vi "Controllo coppia.vi"(0 "C attuale":dbl, 1 "fine rampa C in":bool, 2 "Tutti i dati":T2, 3 "Coppia":T8, 4 "Cmax RPMmax\n inverter":cluster{"Vel max(RPM)":dbl, "Cmax (nm)":dbl}, 5 "RPM PROVA":refnum<vi>, 6 "Coppia letta tors":dbl, 7 "Reset comp":bool, 8 "COPPIA DI FRENATURA [Nm]":refnum<vi>, 9 "Forza controllo vel":bool, 10 "Set C":dbl, 11 "Fine rampa F":bool, 12 "Cmax":dbl, 13 "LOOP TIME (ms)":u32) -> (14 "fine rampa C out":bool, 15 "C stabile":bool, 16 "Set C out":dbl, 17 "Out C":dbl, 18 "Tempo rampa (s)":dbl)   [LabVIEW 2019]
uses:
  cDAQ_PLC Folder/cDAQ/AO List.ctl
  cDAQ_PLC Folder/cDAQ/SET SINGLE AO.ctl
  cDAQ_PLC Folder/cDAQ/DO List.ctl
  cDAQ_PLC Folder/cDAQ/SET SINGLE DO.ctl
  Global FINE AVVIO.vi
  Global_Cmecc_RotBlocc.vi
  <vilib>/addons/control/pid/NI_PID_pid.lvlib
  Global set coppia.vi
  Global stato ctrl coppia.vi
  Global prova in corso.vi
  Global_scelta_banco.vi
  Global Stop command.vi
  Global ctrl potenza.vi
  Servo avviamento.vi
  <vilib>/Analysis/NI_AALBase.lvlib
  <vilib>/addons/control/pid/pid.llb/PID (DBL).vi
  <vilib>/Analysis/1siggen.llb/Ramp Pattern by Samples.vi
  cDAQ/LettureCDAQ_PLC.ctl
  controls/statoAO_plc.ctl
  controls/statoDO.ctl
  ST1200_LIST_IO/StatoDO_PLC.ctl
  cDAQ_PLC Folder/controls/StatoAO_cdaq.ctl
  controls/Tutti_i_dati.ctl
panel:
  out "Boolean":bool=TRUE
  out "Ramp":dbl[](array[numeric])
  in  "Periodo set rpm[s] b2":dbl=2.0 format="%#_13g"
  in  "step rpm B2":dbl=0.5 format="%#_13g"
  in  "Nm b2":dbl=2.0 format="%#_13g"
  in  "Precisione b2":dbl=0.2
  in  "Nm b1":dbl=0.015 format="%#_13g"
  in  "Precisione b1":dbl=0.01
  out "s? t:f":string
  in  "PID b2 gains ctrl velocità":T1={"proportional gain (Kc)"=5.0, "integral time (Ti, min)"=0.01, "derivative time (Td, min)"=0.0}
  out "fine rampa":bool
  in  "reinitialize? (F)":bool
  in  "PID b1 gains ctrl velocità":T1={"proportional gain (Kc)"=250.0, "integral time (Ti, min)"=0.003, "derivative time (Td, min)"=0.0} {"derivative time (Td, min)" format="%.3f"; "integral time (Ti, min)" format="%.3f"; "proportional gain (Kc)" format="%.3f"}
  out "x < y?":bool
  out "x > y?":bool
  in  "step rpm B1":dbl=2.0 format="%#_13g"
  in  "max variazione rpm":dbl=2300.0 format="%#_13g"
  in  "Periodo set rpm[s] b1":dbl=0.5 format="%#_13g"
  out "RPM iniziali":dbl
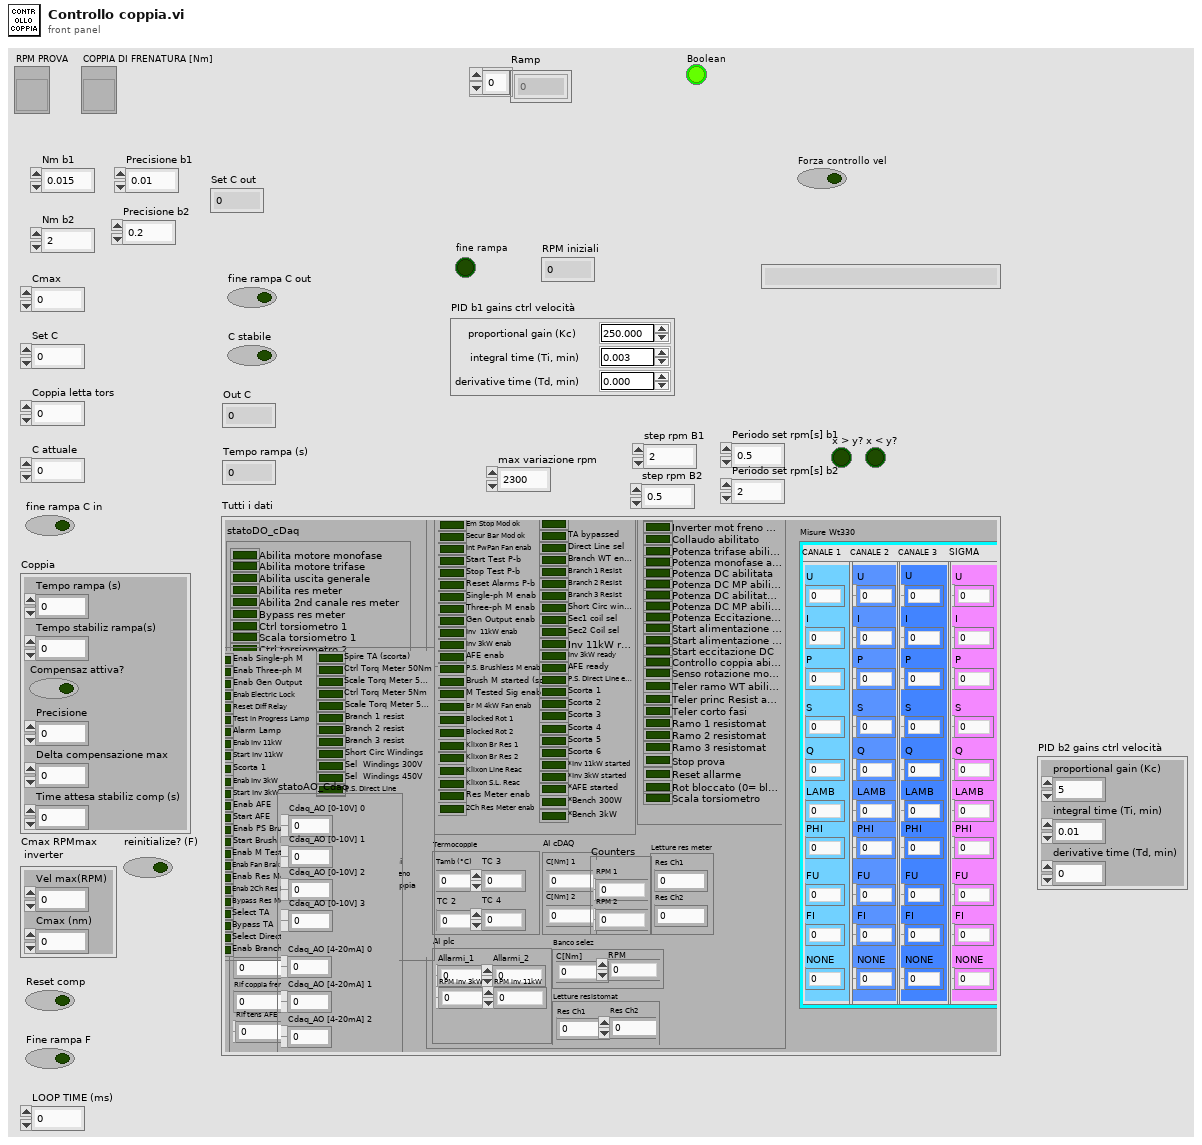
[diagram p1: front panel]
types:
  T1 = cluster{"proportional gain (Kc)":dbl, "integral time (Ti, min)":dbl, "derivative time (Td, min)":dbl}
  T2 = typedef "Tutti_i_dati.ctl" = cluster{"Letture":T3, "Misure Wt330":cluster{"CANALE 1":cluster{"U":dbl, "I":dbl, "P":dbl, "S":dbl, "Q":dbl, "LAMB":dbl, "PHI":dbl, "FU":dbl, "FI":dbl, "NONE":dbl}, "CANALE 2":cluster{"U":dbl, "I":dbl, "P":dbl, "S":dbl, "Q":dbl, "LAMB":dbl, "PHI":dbl, "FU":dbl, "FI":dbl, "NONE":dbl}, "CANALE 3":cluster{"U":dbl, "I":dbl, "P":dbl, "S":dbl, "Q":dbl, "LAMB":dbl, "PHI":dbl, "FU":dbl, "FI":dbl, "NONE":dbl}, "SIGMA":cluster{"U":dbl, "I":dbl, "P":dbl, "S":dbl, "Q":dbl, "LAMB":dbl, "PHI":dbl, "FU":dbl, "FI":dbl, "NONE":dbl}}, "statoAO_PLC":T4, "statoDO_cDaq":T5, "StatoDO_PLC":T6, "statoAO_Cdaq":T7}
  T3 = typedef "LettureCDAQ_PLC.ctl" = cluster{"DI-logici":cluster{"Sistema OK":bool, "Inverter mot freno Run":bool, "Collaudo abilitato":bool, "Potenza trifase abilitata":bool, "Potenza monofase abilitata":bool, "Potenza DC abilitata":bool, "Potenza DC MP abilitata":bool, "Potenza DC abilitata no WT":bool, "Potenza DC MP abilitata no WT":bool, "Potenza Eccitazione abilitata":bool, "Start alimentazione AC":bool, "Start alimentazione DC":bool, "Start eccitazione DC":bool, "Controllo coppia abilitato":bool, "Senso rotazione motore freno":bool, "Teler ramo WT abilitato":bool, "Teler princ Resist abilitato":bool, "Teler corto fasi":bool, "Ramo 1 resistomat":bool, "Ramo 2 resistomat":bool, "Ramo 3 resistomat":bool, "Stop prova":bool, "Reset allarme":bool, "Rot bloccato (0= bloccato)":bool, "Scala torsiometro":bool}, "Termocoppie":cluster{"Tamb (°C)":dbl, "TC 2":dbl, "TC 3":dbl, "TC 4":dbl}, "AI cDAQ":cluster{"C[Nm] 1":dbl, "C[Nm] 2":dbl}, "Counters":cluster{"RPM 1":dbl, "RPM 2":dbl}, "Stato DI_Cdaq":cluster{"Motore monofase abil":bool, "Motore trifase abil":bool, "Uscita generale abil":bool, "2nd ch res meter abil":bool, "TA selezionati":bool, "Pulsante Start prova":bool, "Pulsante Stop prova":bool, "Pulsante Reset allarmi":bool, "Secondari TA aperti":bool, "Res meter abil":bool, "Scorta 1":bool, "Scorta 2":bool, "Scorta 3":bool, "Scorta 4":bool, "Scorta 5":bool, "Scorta 6":bool, "Scorta 7":bool, "Scorta 8":bool, "Scorta 9":bool, "Scorta 10":bool, "Scorta 11":bool, "Scorta 12":bool, "Scorta 13":bool, "Scorta 14":bool, "Scorta 15":bool, "Scorta 16":bool, "Scorta 17":bool, "Scorta 18":bool, "Scorta 19":bool, "Scorta 20":bool, "Scorta 21":bool, "Scorta 22":bool}, "Stato DI_PLC":cluster{"Diff Relay On":bool, "Em Stop Mod ok":bool, "Secur Bar Mod ok":bool, "Int PwPan Fan enab":bool, "Start Test P-b":bool, "Stop Test P-b":bool, "Reset Alarms P-b":bool, "Single-ph M enab":bool, "Three-ph M enab":bool, "Gen Output enab":bool, "Inv  11kW enab":bool, "Inv 3kW enab":bool, "AFE enab":bool, "P.S. Brushless M enab":bool, "Brush M started (scorta)":bool, "M Tested Sig enab":bool, "Br M 4kW Fan enab":bool, "Blocked Rot 1":bool, "Blocked Rot 2":bool, "Klixon Br Res 1":bool, "Klixon Br Res 2":bool, "Klixon Line Reac":bool, "Klixon S.L. Reac":bool, "Res Meter enab":bool, "2Ch Res Meter enab":bool, "Bypass Res Meter":bool, "TA selected":bool, "TA bypassed":bool, "Direct Line sel":bool, "Branch WT enab":bool, "Branch 1 Resist":bool, "Branch 2 Resist":bool, "Branch 3 Resist":bool, "Short Circ windings":bool, "Sec1 coil sel":bool, "Sec2 Coil sel":bool, "Inv 11kW ready":bool, "Inv 3kW ready":bool, "AFE ready":bool, "P.S. Direct Line enab":bool, "Scorta 1":bool, "Scorta 2":bool, "Scorta 3":bool, "Scorta 4":bool, "Scorta 5":bool, "Scorta 6":bool, "*Inv 11kW started":bool, "*Inv 3kW started":bool, "*AFE started":bool, "*Bench 300W":bool, "*Bench 3kW":bool}, "Letture res meter":cluster{"Res Ch1":dbl, "Res Ch2":dbl}, "Banco selez":cluster{"C[Nm]":dbl, "RPM":dbl}, "AI plc":cluster{"Allarmi_1":dbl, "Allarmi_2":dbl, "RPM inv 3kW":dbl, "RPM inv 11kW":dbl}, "Letture resistomat":cluster{"Res Ch1":dbl, "Res Ch2":dbl}}
  T4 = typedef "statoAO_plc.ctl" = cluster{"Rif vel freno":dbl, "Rif coppia freno":dbl, "Rif tens AFE":dbl, "Rif freq AFE":dbl}
  T5 = typedef "statoDO.ctl" = cluster{"Abilita motore monofase":bool, "Abilita motore trifase":bool, "Abilita uscita generale":bool, "Abilita res meter":bool, "Abilita 2nd canale res meter":bool, "Bypass res meter":bool, "Ctrl torsiometro 1":bool, "Scala torsiometro 1":bool, "Ctrl torsiometro 2":bool, "Scala torsiometro 2":bool, "Seleziona TA":bool, "Seleziona linea diretta":bool, "Seleziona spire TA":bool, "Bypass TA":bool, "Lampada Test in progress":bool, "Lampada allarme":bool, "Apri TA secondari":bool, "Scorta 1":bool, "Scorta 2":bool, "Scorta 3":bool, "Scorta 4":bool, "Scorta 5":bool, "Scorta 6":bool, "Scorta 7":bool, "Scorta 8":bool, "Scorta 9":bool, "Scorta 10":bool, "Scorta 11":bool, "Scorta 12":bool, "Scorta 13":bool, "Scorta 14":bool, "Scorta 15":bool}
  T6 = typedef "StatoDO_PLC.ctl" = cluster{"Enab Single-ph M":bool, "Enab Three-ph M":bool, "Enab Gen Output":bool, "Enab Electric Lock":bool, "Reset Diff Relay":bool, "Test in Progress Lamp":bool, "Alarm Lamp":bool, "Enab Inv 11kW":bool, "Start Inv 11kW":bool, "Scorta 1":bool, "Enab Inv 3kW":bool, "Start Inv 3kW":bool, "Enab AFE":bool, "Start AFE":bool, "Enab PS Brush M":bool, "Start Brush M (scorta)":bool, "Enab M Tested Sig":bool, "Enab Fan Brak M 4kW":bool, "Enab Res Meter":bool, "Enab 2Ch Res Meter":bool, "Bypass Res Meter":bool, "Select TA":bool, "Bypass TA":bool, "Select Direct Line":bool, "Enab Branch WT":bool, "Spire TA (scorta)":bool, "Ctrl Torq Meter 50Nm":bool, "Scale Torq Meter 50Nm ":bool, "Ctrl Torq Meter 5Nm":bool, "Scale Torq Meter 5Nm":bool, "Branch 1 resist":bool, "Branch 2 resist":bool, "Branch 3 resist":bool, "Short Circ Windings":bool, "Sel  Windings 300V":bool, "Sel  Windings 450V":bool, "P.S. Direct Line":bool, "Scorta 2":bool, "Scorta 3":bool, "Scorta 4":bool, "Scorta 5":bool, "Scorta 6":bool, "*Reset Allarmi":bool, "*Senso Rotaz freno":bool, "*Controllo Coppia":bool, "*Abilita freno":bool, "*Marcia freno":bool, "*Watch dog":bool, "*Bench 300W":bool, "*Bench 3kW":bool}
  T7 = typedef "StatoAO_cdaq.ctl" = cluster{"Cdaq_AO [0-10V] 0":dbl, "Cdaq_AO [0-10V] 1":dbl, "Cdaq_AO [0-10V] 2":dbl, "Cdaq_AO [0-10V] 3":dbl, "Cdaq_AO [4-20mA] 0":dbl, "Cdaq_AO [4-20mA] 1":dbl, "Cdaq_AO [4-20mA] 2":dbl, "Cdaq_AO [4-20mA] 3":dbl, "Cdaq_AO [4-20mA] 4":dbl, "Cdaq_AO [4-20mA] 5":dbl, "Cdaq_AO [4-20mA] 6":dbl, "Cdaq_AO [4-20mA] 7":dbl}
  T8 = cluster{"Tempo rampa (s)":dbl, "Tempo stabiliz rampa(s)":dbl, "Compensaz attiva?":bool, "Precisione":dbl, "Delta compensazione max":dbl, "Time attesa stabiliz comp (s)":dbl}
  T9 = typedef "SET SINGLE AO.ctl" = cluster{"AO":T10, "Value":dbl}
  T10 = typedef "AO List.ctl" = enum16{"OFF: ALL AO", "Vout Variac", "Vout Freq", "Vout 3", "Vout 4", "Forza AO", "*V eccitazion", "*I eccitazione", "*Rif vel inv freno", "*Rif coppia inv freno", "Exit"}
  T11 = enum8{"Enabled", "Disabled", "Disabled and Grayed Out"}
  T12 = typedef "SET SINGLE DO.ctl" = cluster{"DO":T13, "Value":bool}
  T13 = typedef "DO List.ctl" = enum16{"OFF: ALL DO", "Seleziona banco 1", "Seleziona banco 2", "Reset allarmi", "*Start inverter motore freno", "*Senso rotaz motore freno", "*Abilitazione controllo coppia", "Bypass res meter", "Telerutt scelta linea 60A", "Telerutt scelta spire 50A", "Scelta TA", "Bypass TA", "*Abilit teler ramo WT", "*Abil teler ramo princ Resist", "*Abil teler ramo 1 Resist", "*Abil teler ramo 2 Resist", "*Abil teler ramo 3 Resist", "*Abil cortocirc avvolgim", "*Controllo torsiometro", "*Scala torsiometro", "Collaudo in corso", "*Allarme presente", "Abilita piattaf (0=abil)", "Abilitazione elettroserratura", "Exit", "*Abilita collaudo", "*Abilita potenza trifase", "*Abilita potenza monofase", "*Abilita potenza DC", "*Abilita potenza DC no WT", "*Abilita potenza DC MP", "*Abilita potenza DC MP no WT", "*Start Alimentazione AC", "*Start Alimentazione DC", "*Start eccitazione DC", "*Disabilita teleruttori potenza", "Set teleruttori prova a freddo", "Watchdog", "Forza DO", "*Abil teler ramo princ ResistMeter", "Abil AFE rigenerativo"}
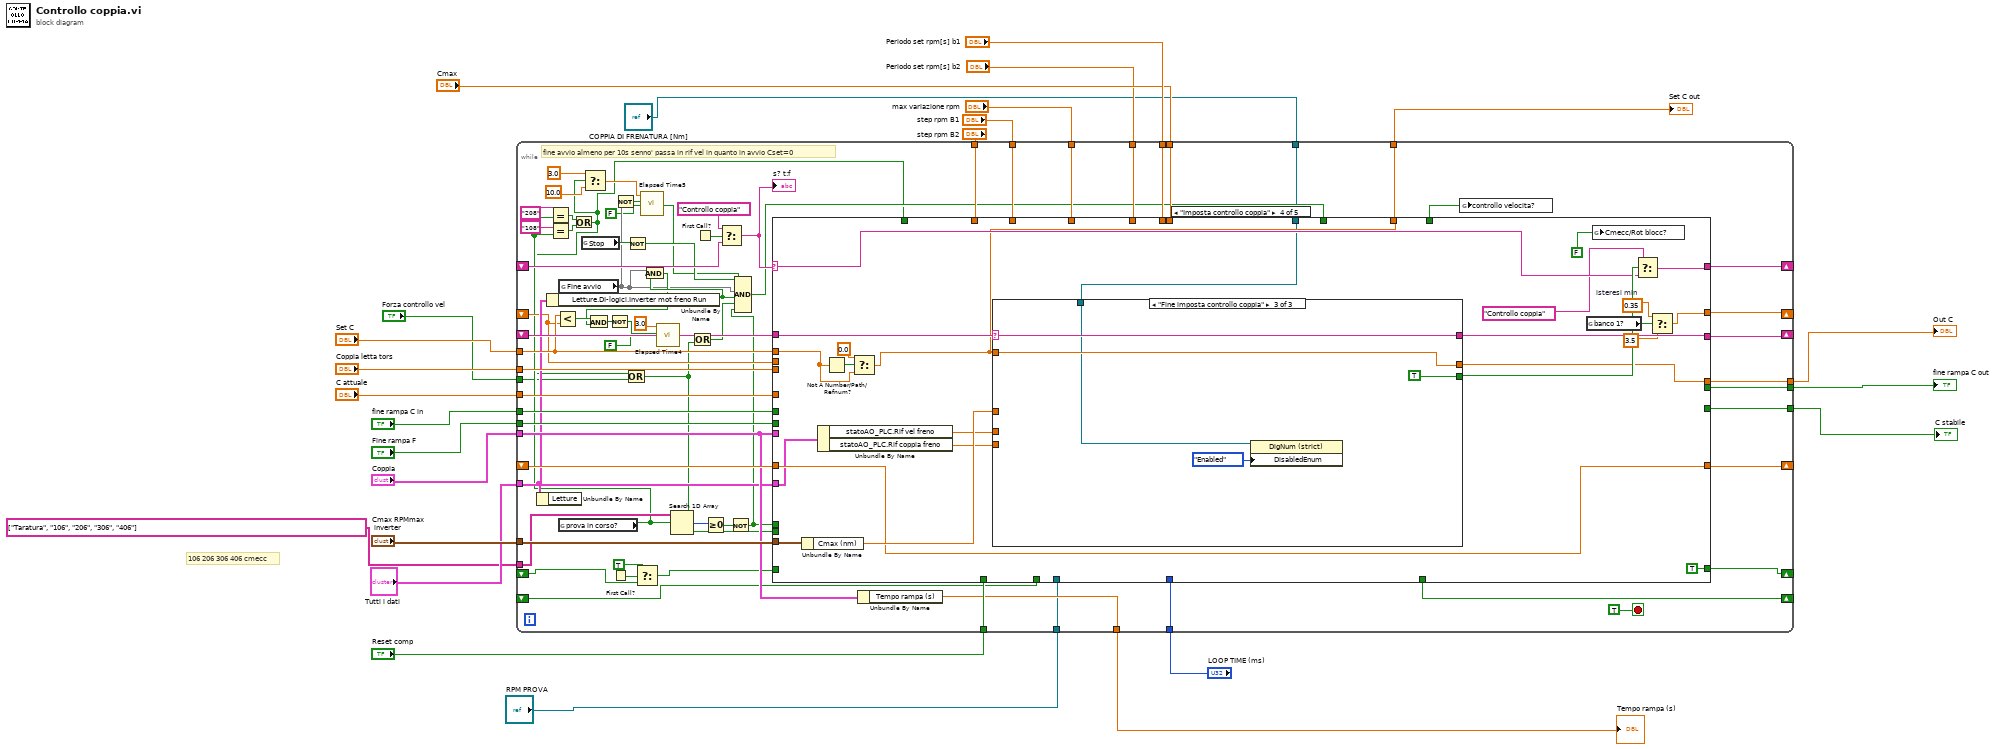
[diagram p0: block diagram]
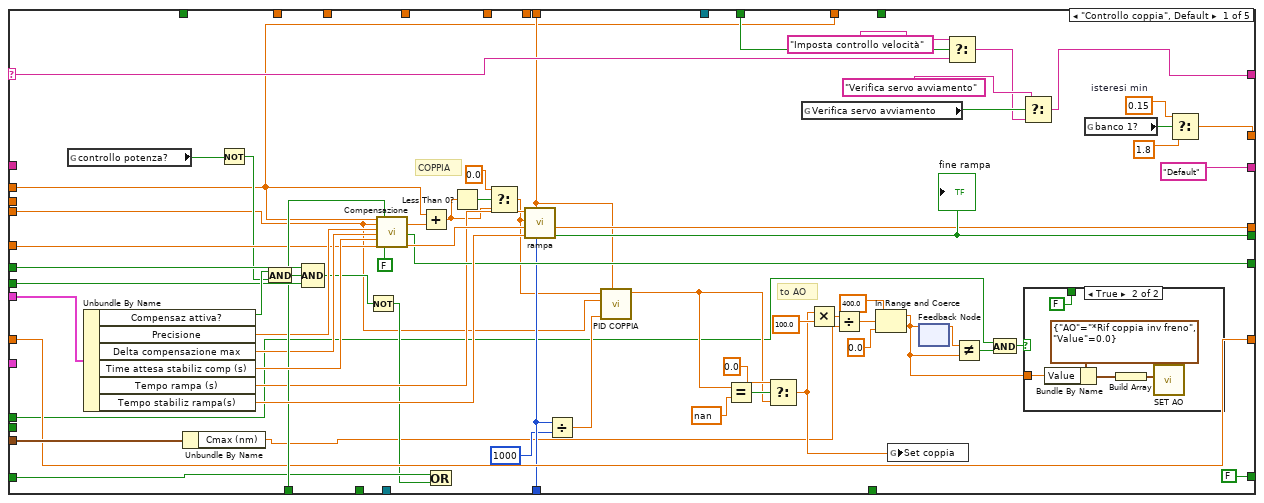
[diagram p2: hidden frame]
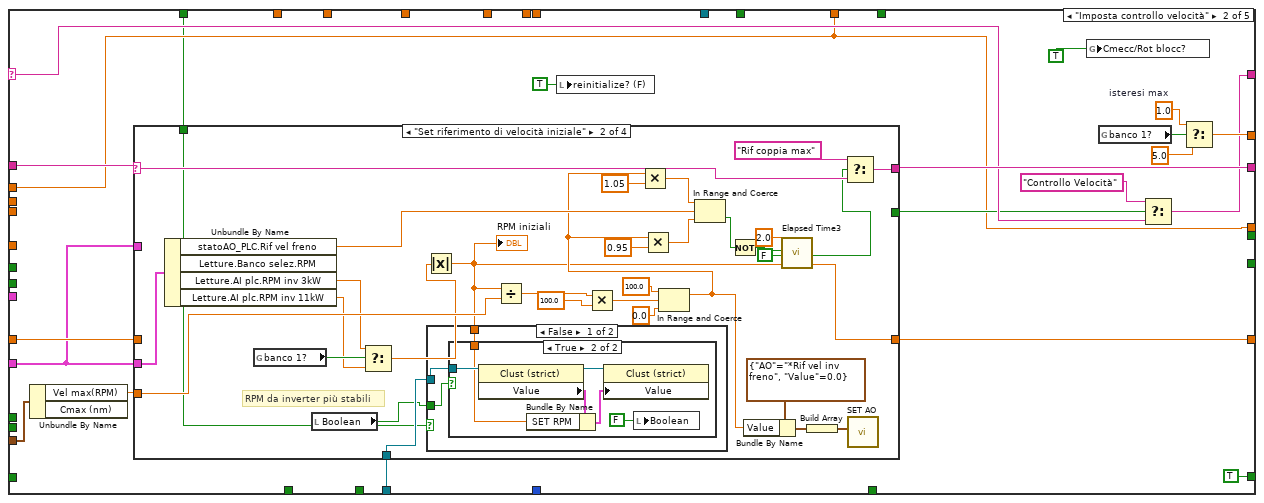
[diagram p4: hidden frame]
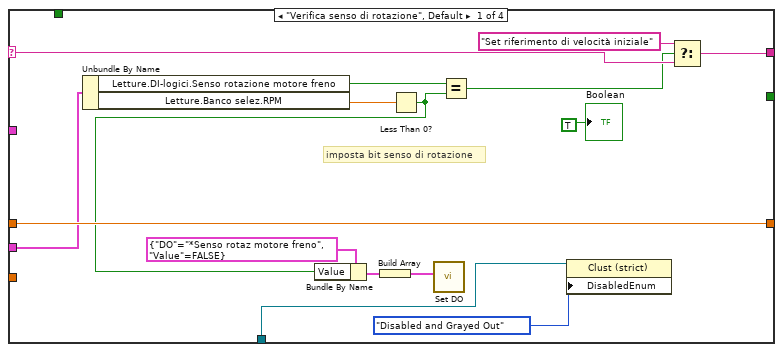
[diagram p5: hidden frame]
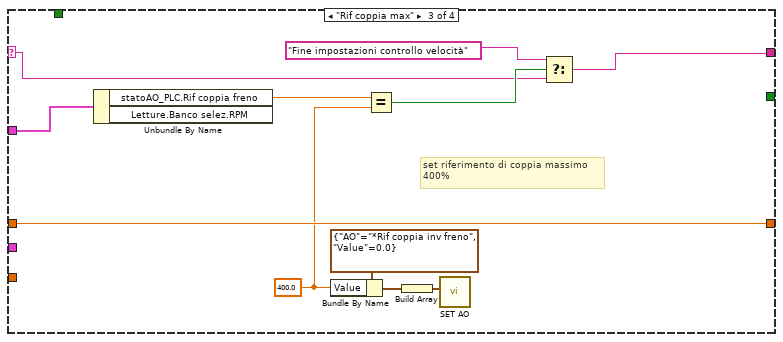
[diagram p8: hidden frame]
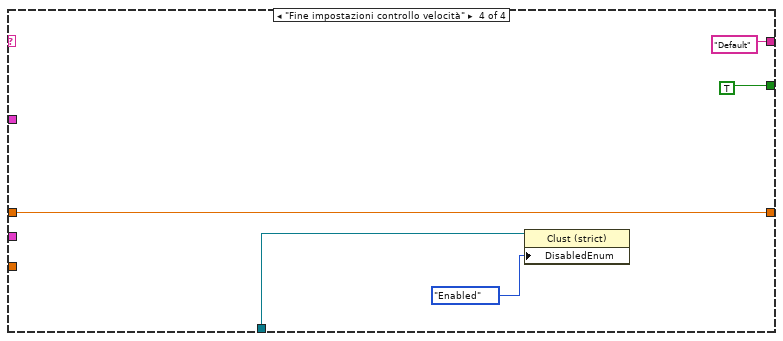
[diagram p9: hidden frame]
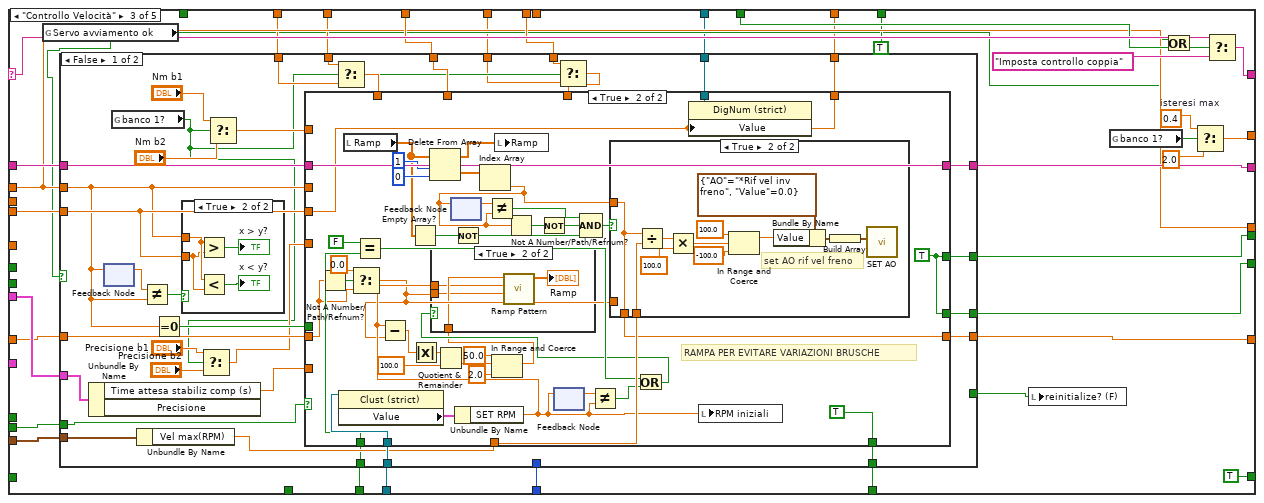
[diagram p10: hidden frame]
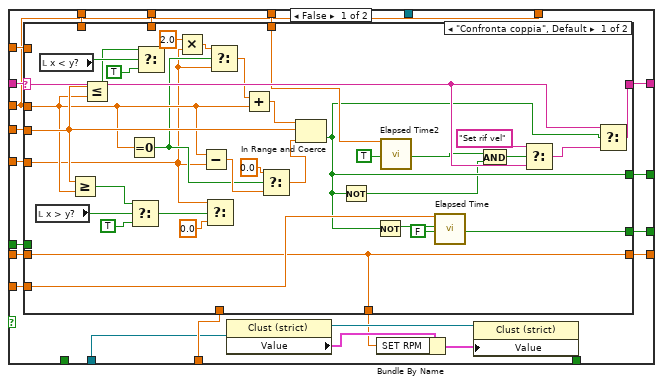
[diagram p11: hidden frame]
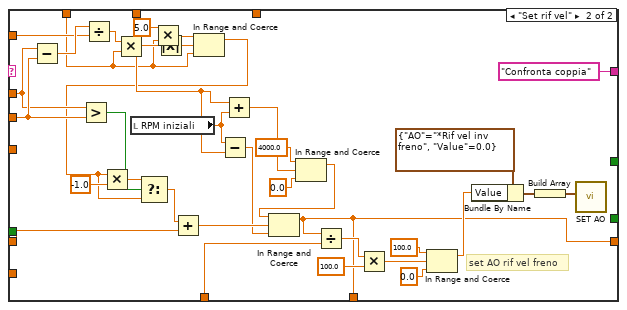
[diagram p12: hidden frame]
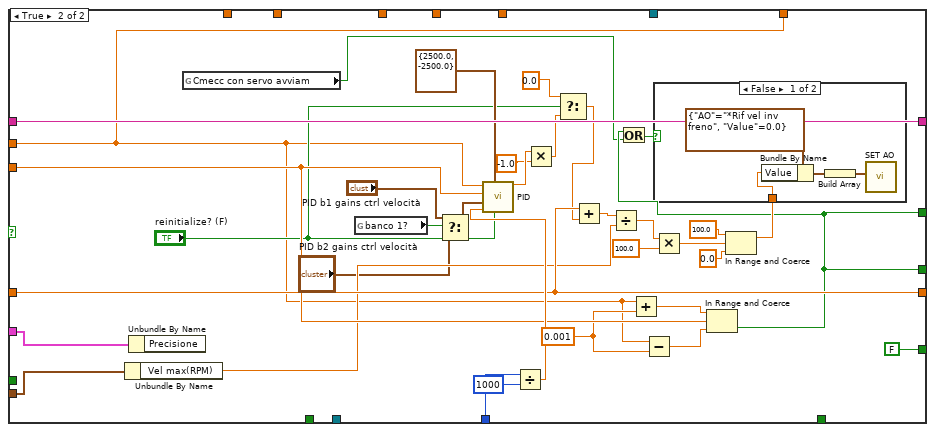
[diagram p16: hidden frame]
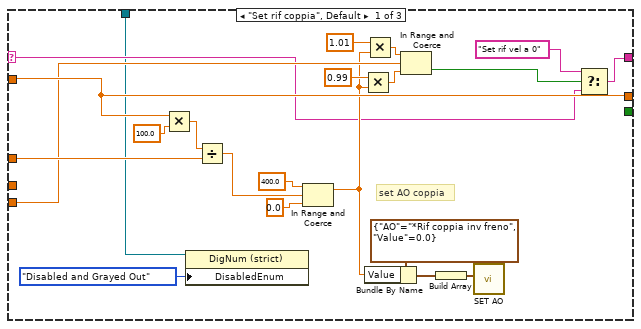
[diagram p18: hidden frame]
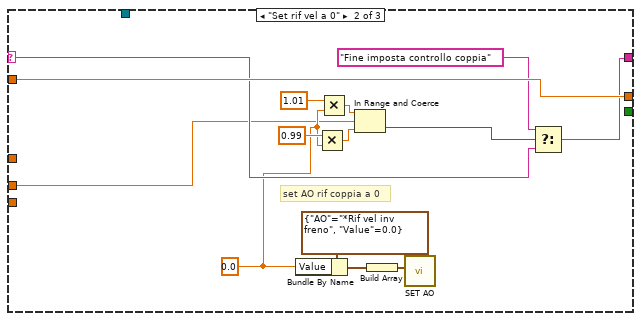
[diagram p19: hidden frame]
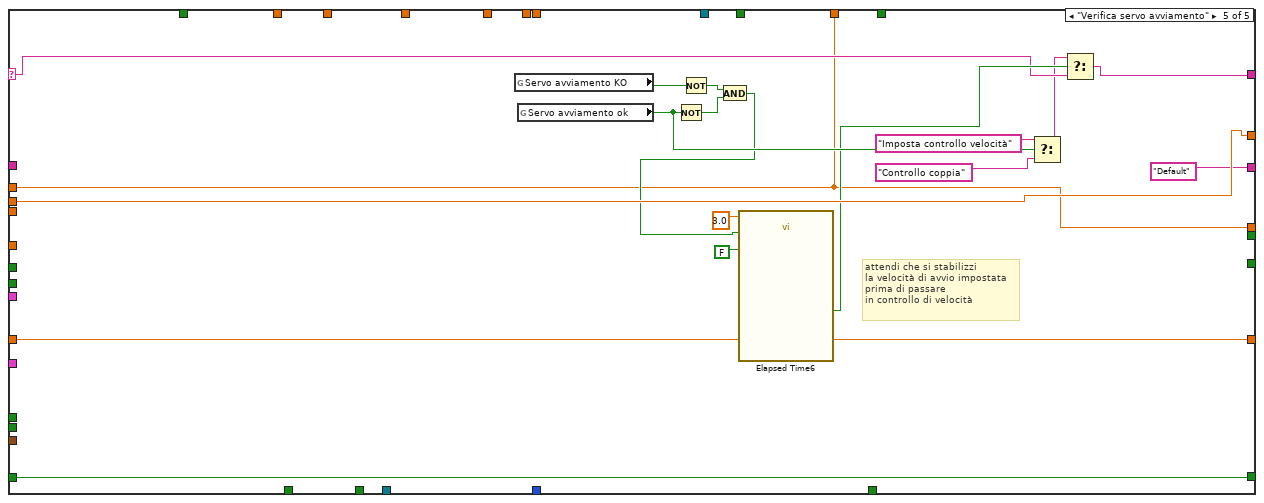
[diagram p20: hidden frame]
diagram:
  # "106 206 306 406 cmecc"
  n1 = while {
    tunnel: "LOOP TIME (ms)" -> [w99]
    tunnel: "C attuale" -> [w98]
    tunnel: "Coppia" -> [w79]
    tunnel: "fine rampa C in" -> [w97]
    tunnel: "Fine rampa F" -> [w96]
    tunnel: "Reset comp" -> [w95]
    tunnel: "Coppia letta tors" -> [w94]
    tunnel: "Set C" -> [w75]
    tunnel: [w93] -> w22
    tunnel: [w92] -> w23
    tunnel: [w78] -> w24
    tunnel: "Cmax RPMmax\n inverter" -> [w91]
    tunnel: [w90] -> w14
    tunnel: "Cmax" -> [w89]
    shift-right: [w87] -> _
    shift-left: _ -> [w77]
    shift-right: [w85] -> _
    shift-left: _ -> [w86]
    tunnel: "Tutti i dati" -> [w70]
    shift-right: [w84] -> _
    shift-left: _ -> [w83]
    tunnel: "max variazione rpm" -> [w82]
    tunnel: "step rpm B1" -> [w81]
    tunnel: "Periodo set rpm[s] b1" -> [w80]
    tunnel: string[] ["Taratura", "106", "206", "306", "406"] -> [w69]
    shift-right: [w61] -> _
    shift-left: _ -> [w47]
    shift-right: [w55] -> _
    shift-left: _ -> [w53]
    tunnel: "step rpm B2" -> [w50]
    tunnel: "Periodo set rpm[s] b2" -> [w45]
    tunnel: "Forza controllo vel" -> [w29]
    tunnel: "RPM PROVA" -> [w41]
    tunnel: [w40] -> w3
    shift-right: [w39] -> _
    shift-left: _ -> [w38]
    tunnel: "COPPIA DI FRENATURA [Nm]" -> [w26]
    stop <- TRUE stop-if-true
    # "fine avvio almeno per 10s senno' passa in rif vel in quanto in avvio Cset=0"
    n2 = Unbundle By Name(w70) -> ()  [unwired: 1 out]
    n3 = Unbundle By Name(w70) -> ("Letture.DI-logici.Inverter mot freno Run"=w64:bool)
    n4 = Less?(x=w75, y=w47) -> (x < y?=w73:bool)
    n5 = global read "Global prova in corso.vi" "prova in corso?"() -> (w34:bool)
    n6 = Equal?(x=w34, y="208") -> (x = y?=w30:bool)
    n7 = Equal?(x="108", y=w34) -> (x = y?=w31:bool)
    n8 = global read "Global fine avvio.vi" "Fine avvio"() -> (w60)
    n9 = Or(x=w30, y=w31) -> (x .or. y?=w27:bool)
    n10 = global read "Global Stop command.vi" "Stop"() -> (w66:bool)
    n11 = Select(t=3.0, s=w27, f=10.0 ("Time Target (s)")) -> (s? t:f=w36:dbl)
    n12 = First Call?() -> (First Call?: T/F=w54:bool)
    n13 = Not(x=w60) -> (.not. x?=w59:bool)
    n14 = Or(x=w27, y=w29) -> (x .or. y?=w28:bool)
    n15 = Not(x=w66) -> (.not. x?=w65:bool)
    n16 = Select(t=TRUE, s=w54, f=w53) -> (s? t:f=w52:bool)
    n17 = call "Elapsed Time5"("Time Target (s)"=w36, "Reset"=w59, "Auto Reset"=FALSE) -> ("Time has Elapsed"=w57:bool)  [unwired: 9 in, 7 out]
    n18 = And(x=w60, y=w64) -> (x .and. y?=w62:bool)
    n19 = And(x=w73, y=w62) -> (x .and. y?=w63:bool)
    n20 = Not(x=w63) -> (.not. x?=w72:bool)
    n21 = call "Elapsed Time4"("Time Target (s)"=3.0, "Reset"=w72, "Auto Reset"=FALSE) -> ("Time has Elapsed"=w43:bool)  [unwired: 9 in, 7 out]
    n22 = Search 1D Array(1D array=w69, element=w34) -> (index of element=w68:i32)  [unwired: 1 in]
    n23 = Or(x=w43, y=w28) -> (x .or. y?=w42:bool)
    n24 = First Call?() -> (First Call?: T/F=w56:bool)
    n25 = Greater Or Equal To 0?(x=w68) -> (x >= 0?=w67:bool)
    n26 = Select(t="Controllo coppia", s=w56, f=w77) -> (s? t:f=w48:string)
    "s? t:f" <- w48
    n27 = Not(x=w67) -> (.not. x?=w46:bool)
    n28 = Compound Arithmetic op=AND(w57, w65, w60, w64, w42, w46) -> (w44:bool)
    n29 = case shown="\"Imposta controllo coppia\"" w48 {
      selector: w48 -> [w139 w187 w292 w540 w589]
      tunnel: w99 -> [w134 _ w280 _ _]
      tunnel: w98 -> [w129 _ _ _ _]
      tunnel: w79 -> [w159 _ w290 _ _]
      tunnel: w97 -> [w158 _ _ _ _]
      tunnel: w96 -> [w156 _ _ _ _]
      tunnel: w95 -> [w155 _ _ _ _]
      tunnel: w94 -> [w111 _ w281 _ _]
      tunnel: w75 -> [w100 w170 w282 w524 w587]
      tunnel: [w132 _ w284 _ _] -> w93
      tunnel: [w153 _ w285 _ _] -> w92
      tunnel: w91 -> [w148 w185 w287 w544 _]
      tunnel: [w112 w170 w282 w537 w587] -> w90
      tunnel: w89 -> [w101 _ _ _ _]
      tunnel: [w104 w172 w293 w539 w595] -> w87
      tunnel: w44 -> [w138 _ w291 _ _]
      tunnel: w86 -> [_ w189 w296 w545 _]
      tunnel: ["Default" w188 w295 w542 "Default"] -> w85
      tunnel: w70 -> [_ w180 _ w534 _]
      tunnel: [w135 w182 w288 w536 w604] -> w84
      tunnel: w83 -> [w135 w181 w289 w536 w604]
      tunnel: w82 -> [_ _ w286 _ _]
      tunnel: w81 -> [_ _ w272 _ _]
      tunnel: w80 -> [_ _ w283 _ _]
      tunnel: [_ _ TRUE _ _] -> w76
      tunnel: [w125 w174 w275 w529 w602] -> w61
      tunnel: [FALSE TRUE TRUE TRUE w603] -> w55
      tunnel: w52 -> [w117 _ _ _ w603]
      tunnel: w50 -> [_ _ w271 _ _]
      tunnel: w47 -> [_ _ _ _ w602]
      tunnel: w46 -> [w102 _ _ _ _]
      tunnel: w45 -> [_ _ w268 _ _]
      tunnel: w41 -> [_ w171 w266 _ _]
      tunnel: w28 -> [_ _ w267 _ _]
      tunnel: [w100 w170 w265 w523 w587] -> w40
      tunnel: [_ _ w264 _ _] -> w39
      tunnel: w38 -> [_ _ w263 _ _]
      tunnel: w27 -> [_ w169 _ _ _]
      tunnel: w26 -> [_ _ w262 w522 _]
      frame "Controllo coppia", Default {
        w128 = 0.15  # isteresi min
        # "to AO"
        # "COPPIA"
        n30 = global read "Global ctrl potenza.vi" "controllo potenza?"() -> (w116:bool)
        n31 = Unbundle By Name(w159) -> ("Compensaz attiva?"=w157:bool, "Precisione"=w154:dbl, "Delta compensazione max"=w131:dbl, "Time attesa stabiliz comp (s)"=w160:dbl, "Tempo rampa (s)"=w151:dbl, "Tempo stabiliz rampa(s)"=w161:dbl)
        n32 = Unbundle By Name(w148) -> ("Cmax (nm)"=w113:dbl)
        n33 = Not(x=w116) -> (.not. x?=w123:bool)
        n34 = And(x=w157, y=w123) -> (x .and. y?=w124:bool)
        n35 = Compound Arithmetic op=AND(w158, w124, w156) -> (w115:bool)
        n36 = Not(x=w115) -> (.not. x?=w114:bool)
        n37 = call "Compensazione.vi"("Grandezza target"=w100, "Grandezza reale letta"=w111, "Precisione"=w154, "Delta compensazione max"=w131, "Time attesa stabilizzazione (s)"=w160, "Grandezza attuale in"=w129, "Reset comp?"=w155, "Compensazione abilitata"=FALSE) -> ("compensazione"=w162:dbl, "Grandezza stabilizz?"=w153:bool, "Grandezza attuale out"=w163:dbl)  [unwired: 9 in]
        n38 = Add(x=w100, y=w162) -> (x+y=w142:dbl)
        n39 = Or(x=w117, y=w114) -> ()  [unwired: 1 out]
        n40 = Less Than 0?(x=w142) -> (x < 0?=w143:bool)
        n41 = Select(t=0.0, s=w143, f=w142) -> (s? t:f=w108:dbl)
        n42 = call "rampa.vi"("tempo ciclo (ms)"=w134, "Valore massimo"=w101, "Tempo di stabilizzazione (s)"=w161, "reale"=w163, "set"=w108, "tempo rampa (s)"=w151) -> ("fine rampa"=w132:bool, "OUT"=w112:dbl)  [unwired: 4 in]
        "fine rampa" <- w132
        n43 = Divide(x=w134, y=u32 1000) -> (x/y=w109:dbl)
        n44 = call "PID COPPIA.vi"("Cmax"=w101, "dt (s)"=w109, "process variable"=w111, "setpoint"=w108) -> ("output"=w110:dbl)  [unwired: 7 in]
        n45 = Equal?(x=w110, y=nan) -> (x = y?=w122:bool)
        n46 = Select(t=0.0, s=w122, f=w110) -> (s? t:f=w119:dbl)
        n47 = global read "Servo avviamento.vi" "Verifica servo avviamento"() -> (w107:bool)
        n48 = Multiply(x=w119, y=100.0) -> (x*y=w152:dbl)
        n49 = Divide(x=w152, y=w113) -> (x/y=w150:dbl)
        n50 = In Range and Coerce(upper limit=400.0, x=w150, lower limit=0.0) -> (coerced(x)=w145:dbl)  [unwired: 1 out]
        n51 = global write "Global set coppia.vi" "Set coppia"(w119) -> ()
        n52 = feedback #1() -> (w146:dbl)  [unwired: 1 in]
        n53 = feedback-in #1(w145) -> ()
        n54 = Select(t="Imposta controllo velocità", s=w138, f=w139) -> (s? t:f=w105:string)
        n55 = Not Equal?(x=w146, y=w145) -> (x != y?=w147:bool)
        n56 = And(x=w102, y=w147) -> (x .and. y?=w103:bool)
        n57 = Select(t="Verifica servo avviamento", s=w107, f=w105) -> (s? t:f=w104:string)
        n58 = case shown="True" w103 {
          tunnel: w145 -> [_ w168]
          tunnel: [_ FALSE ("reinitialize? (F) 2")] -> _
          frame False {
          }
          frame True {
            n59 = Bundle By Name(cluster=T9 {"AO"=enum."*Rif coppia inv freno", "Value"=0.0} ("Cluster SET AO"), "Value"=w168) -> (w166:T9)
            n60 = Build Array(w166) -> (w164:T9[])
            n61 = call "SET AO.vi"("Cluster SET AO"=w164) -> ()  [unwired: 10 in, 1 out]
          }
        }
        n62 = global read "Global_scelta_banco.vi" "banco 1?"() -> (w127:bool)
        n63 = Select(t=w128, s=w127, f=1.8) -> (s? t:f=w125:dbl)
      }
      frame "Imposta controllo velocità" {
        w177 = 1.0  # isteresi max
        n64 = Unbundle By Name(w185) -> ("Vel max(RPM)"=w184:dbl)  [unwired: 1 out]
        n65 = case shown="\"Set riferimento di velocità iniziale\"" w189 {
          selector: w189 -> [w204 w232 w248 _]
          tunnel: [w203 w231 w246 "Default" ("t")] -> w188
          tunnel: w180 -> [w195 w233 _ _]
          tunnel: w184 -> [_ w234 _ _]
          tunnel: [_ _ _ TRUE] -> w183
          tunnel: [w201 w207 w253 w259] -> w182
          tunnel: w181 -> [w201 _ w253 w259]
          tunnel: w180 -> [_ _ w252 _]
          tunnel: w171 -> [w191 w208 _ w257]
          tunnel: w169 -> [_ w206 _ _]
          frame "Verifica senso di rotazione", Default {
            # "imposta bit senso di rotazione"
            n66 = Unbundle By Name(w195) -> ("Letture.DI-logici.Senso rotazione motore freno"=w200:bool, "Letture.Banco selez.RPM"=w199:dbl)
            n67 = Less Than 0?(x=w199) -> (x < 0?=w193:bool)
            n68 = Bundle By Name(cluster=T12 {"DO"=enum."*Senso rotaz motore freno", "Value"=FALSE} ("Cluster SET DO"), "Value"=w193) -> (w197:T12)
            n69 = Build Array(w197) -> (w196:T12[])
            n70 = call "Set DO.vi"("Cluster SET DO"=w196) -> ()  [unwired: 10 in, 1 out]
            n71 = Equal?(x=w200, y=w193) -> (x = y?=w194:bool)
            n72 = property class="Clust (strict)"(reference=w191, "DisabledEnum"=T11."Disabled and Grayed Out" ("Disabled")) -> ()  [unwired: 1 in, 2 out]
            n73 = Select(t="Set riferimento di velocità iniziale", s=w194, f=w204) -> (s? t:f=w203:string)
            "Boolean" <- TRUE
          }
          frame "Set riferimento di velocità iniziale" {
            # "RPM da inverter più stabili"
            n74 = Unbundle By Name(w233) -> ("statoAO_PLC.Rif vel freno"=w219:dbl, "Letture.AI plc.RPM inv 3kW"=w211:dbl, "Letture.AI plc.RPM inv 11kW"=w210:dbl)  [unwired: 1 out]
            n75 = global read "Global_scelta_banco.vi" "banco 1?"() -> (w212:bool)
            n76 = local read "Boolean"() -> (w205:bool)
            n77 = Select(t=w211, s=w212, f=w210) -> (s? t:f=w209:dbl)
            n78 = Absolute Value(x=w209) -> (abs(x)=w207:dbl)
            "RPM iniziali" <- w207
            n79 = case shown="False" w206 {
              tunnel: w208 -> [w239 _]
              tunnel: w207 -> [w238 _]
              tunnel: w205 -> [w237 _]
              frame False {
                n80 = case shown="True" w237 {
                  tunnel: w239 -> [_ w242]
                  tunnel: w238 -> [_ w241]
                  frame False {
                  }
                  frame True {
                    n81 = property class="Clust (strict)"(reference=w242) -> (reference out=w244:refnum<vi>, "Value"=w245:cluster{"SET RPM":dbl, "SENSO ROT.":bool})  [unwired: 1 in, 1 out]
                    n82 = Bundle By Name(cluster=w245, "SET RPM"=w241) -> (w243:cluster{"SET RPM":dbl, "SENSO ROT.":bool})
                    n83 = property class="Clust (strict)"(reference=w244, "Value"=w243) -> ()  [unwired: 1 in, 2 out]
                    n84 = local write "Boolean"(FALSE ("Boolean")) -> ()
                  }
                }
              }
              frame True {
              }
            }
            n85 = Divide(x=w207, y=w234) -> (x/y=w235:dbl)
            n86 = Multiply(x=w235, y=100.0) -> (x*y=w228:dbl)
            n87 = In Range and Coerce(upper limit=100.0, x=w228, lower limit=0.0) -> (coerced(x)=w218:dbl)  [unwired: 1 out]
            n88 = Multiply(x=w218, y=1.05) -> (x*y=w221:dbl)
            n89 = Multiply(x=w218, y=0.95) -> (x*y=w223:dbl)
            n90 = In Range and Coerce(upper limit=w221, x=w219, lower limit=w223) -> (In Range?=w217:bool)  [unwired: 1 out]
            n91 = Not(x=w217) -> (.not. x?=w216:bool)
            n92 = Bundle By Name(cluster=T9 {"AO"=enum."*Rif vel inv freno", "Value"=0.0} ("Cluster SET AO"), "Value"=w218) -> (w225:T9)
            n93 = call "Elapsed Time3"("Time Target (s)"=2.0, "Reset"=w216, "Auto Reset"=FALSE) -> ("Time has Elapsed"=w214:bool)  [unwired: 9 in, 7 out]
            n94 = Build Array(w225) -> (w226:T9[])
            n95 = Select(t="Rif coppia max", s=w214, f=w232) -> (s? t:f=w231:string)
            n96 = call "SET AO.vi"("Cluster SET AO"=w226) -> ()  [unwired: 10 in, 1 out]
          }
          frame "Rif coppia max" {
            w250 = 400.0 ("upper limit")
            # "set riferimento di coppia massimo\n400%"
            n97 = Unbundle By Name(w252) -> ("statoAO_PLC.Rif coppia freno"=w251:dbl)  [unwired: 1 out]
            n98 = Bundle By Name(cluster=T9 {"AO"=enum."*Rif coppia inv freno", "Value"=0.0} ("Cluster SET AO"), "Value"=w250) -> (w256:T9)
            n99 = Equal?(x=w251, y=w250) -> (x = y?=w249:bool)
            n100 = Build Array(w256) -> (w254:T9[])
            n101 = call "SET AO.vi"("Cluster SET AO"=w254) -> ()  [unwired: 10 in, 1 out]
            n102 = Select(t="Fine impostazioni controllo velocità", s=w249, f=w248) -> (s? t:f=w246:string)
          }
          frame "Fine impostazioni controllo velocità" {
            n103 = property class="Clust (strict)"(reference=w257, "DisabledEnum"=T11."Enabled" ("Disabled")) -> ()  [unwired: 1 in, 2 out]
          }
        }
        n104 = local write "reinitialize? (F)"(TRUE ("reinitialize? (F)")) -> ()
        n105 = global write "Global_Cmecc_RotBlocc.vi" "Cmecc/Rot blocc?"(TRUE ("Cmecc/Rot blocc?")) -> ()
        n106 = global read "Global_scelta_banco.vi" "banco 1?"() -> (w176:bool)
        n107 = Select(t="Controllo Velocità", s=w183, f=w187) -> (s? t:f=w172:string)
        n108 = Select(t=w177, s=w176, f=5.0) -> (s? t:f=w174:dbl)
      }
      frame "Controllo Velocità" {
        w277 = 0.4  # isteresi max
        n109 = global read "Servo avviamento.vi" "Servo avviamento ok"() -> (w269:bool)
        n110 = case shown="False" w269 {
          tunnel: w296 -> [w331 w517]
          tunnel: [w330 w517] -> w295
          tunnel: w290 -> [w329 w511]
          tunnel: w289 -> [w328 w507]
          tunnel: [w327 w507] -> w288
          tunnel: w287 -> [w326 w501]
          tunnel: w286 -> [w325 _]
          tunnel: [w323 w488] -> w285
          tunnel: [w322 w488] -> w284
          tunnel: w283 -> [w306 _]
          tunnel: w282 -> [w315 w483]
          tunnel: w281 -> [w319 w510]
          tunnel: w280 -> [_ w514]
          tunnel: [_ FALSE ("reinitialize? (F)")] -> w278
          tunnel: w272 -> [w310 _]
          tunnel: w271 -> [w309 _]
          tunnel: w268 -> [w304 _]
          tunnel: w267 -> [w303 _]
          tunnel: w266 -> [w302 _]
          tunnel: [w301 w483] -> w265
          tunnel: [w299 _] -> w264
          tunnel: w263 -> [w298 _]
          tunnel: w262 -> [w297 _]
          frame False {
            n111 = Unbundle By Name(w329) -> ("Time attesa stabiliz comp (s)"=w324:dbl)  [unwired: 1 out]
            n112 = feedback #2() -> (w321:dbl)  [unwired: 1 in]
            n113 = feedback-in #2(w315) -> ()
            n114 = global read "Global_scelta_banco.vi" "banco 1?"() -> (w307:bool)
            n115 = Unbundle By Name(w326) -> ("Vel max(RPM)"=w300:dbl)
            n116 = Not Equal?(x=w321, y=w315) -> (x != y?=w320:bool)
            n117 = Equal To 0?(x=w315) -> (x = 0?=w314:bool)
            n118 = case shown="True" w320 {
              tunnel: w315 -> [_ w481]
              tunnel: w319 -> [_ w480]
              frame False {
              }
              frame True {
                n119 = Greater?(x=w481, y=w480) -> (0:→"x > y?":bool)
                n120 = Less?(x=w481, y=w480) -> (x < y?=→"x < y?":bool)
              }
            }
            n121 = Select(t="Precisione b1", s=w307, f="Precisione b2") -> (s? t:f=w311:dbl)
            n122 = Select(t="Nm b1", s=w307, f="Nm b2") -> (s? t:f=w316:dbl)
            n123 = Select(t=w310, s=w307, f=w309) -> (s? t:f=w308:dbl)
            n124 = Select(t=w306, s=w307, f=w304) -> (s? t:f=w305:dbl)
            n125 = case shown="True" w303 {
              tunnel: w331 -> [w352 w462]
              tunnel: [w351 w462] -> w330
              tunnel: w328 -> [w350 w427]
              tunnel: [w349 w436] -> w327
              tunnel: w300 -> [w348 w457]
              tunnel: w325 -> [w347 _]
              tunnel: w324 -> [w346 _]
              tunnel: [w345 w461] -> w323
              tunnel: [w344 w461] -> w322
              tunnel: w319 -> [w343 w423]
              tunnel: w316 -> [w342 _]
              tunnel: w315 -> [w337 _]
              tunnel: w314 -> [w341 _]
              tunnel: w311 -> [w340 _]
              tunnel: w308 -> [w339 _]
              tunnel: w305 -> [w338 _]
              tunnel: w302 -> [w336 w459]
              tunnel: [w337 w423] -> w301
              tunnel: [_ TRUE] -> w299
              tunnel: w298 -> [_ w455]
              tunnel: w297 -> [_ w424]
              frame False {
                n126 = case shown="\"Confronta coppia\", Default" w352 {
                  selector: w352 -> [w379 _]
                  tunnel: w337 -> [w362 w404]
                  tunnel: w343 -> [w370 w405]
                  tunnel: [w386 "Confronta coppia" ("f")] -> w351
                  tunnel: w340 -> [w356 _]
                  tunnel: [w364 _] -> w344
                  tunnel: w350 -> [w353 w422]
                  tunnel: [w353 w387] -> w349
                  tunnel: w348 -> [_ w414]
                  tunnel: w347 -> [_ w409]
                  tunnel: w339 -> [_ w397]
                  tunnel: w346 -> [w385 _]
                  tunnel: [w382 _] -> w345
                  tunnel: w338 -> [w376 _]
                  tunnel: w342 -> [_ w402]
                  tunnel: w341 -> [_ _]
                  tunnel: [w353 w387] -> w332
                  frame "Confronta coppia", Default {
                    n127 = local read "x > y?"() -> (w375:bool)
                    n128 = local read "x < y?"() -> (w368:bool)
                    n129 = Greater Or Equal?(x=w370, y=w362) -> (x >= y?=w373:bool)
                    n130 = Less Or Equal?(x=w370, y=w362) -> (x <= y?=w367:bool)
                    n131 = Equal To 0?(x=w362) -> (x = 0?=w358:bool)
                    n132 = Select(t=w373, s=w375, f=TRUE) -> (s? t:f=w372:bool)
                    n133 = Select(t=w367, s=w368, f=TRUE) -> ()  [unwired: 1 out]
                    n134 = Multiply(x=2.0, y=w356) -> (x*y=w354:dbl)
                    n135 = Subtract(x=w362, y=w356) -> (x-y=w361:dbl)
                    n136 = Select(t=w356, s=w372, f=0.0) -> ()  [unwired: 1 out]
                    n137 = Select(t=w354, s=w358, f=w356) -> (s? t:f=w357:dbl)
                    n138 = Add(x=w357, y=w362) -> (x+y=w366:dbl)
                    n139 = Select(t=0.0, s=w358, f=w361) -> (s? t:f=w359:dbl)
                    n140 = In Range and Coerce(upper limit=w366, x=w370, lower limit=w359) -> (In Range?=w364:bool)  [unwired: 1 out]
                    n141 = Not(x=w364) -> (.not. x?=w363:bool)
                    n142 = Not(x=w364) -> (.not. x?=w384:bool)
                    n143 = call "Elapsed Time2"("Time Target (s)"=w376, "Auto Reset"=TRUE) -> ("Time has Elapsed"=w378:bool)  [unwired: 10 in, 7 out]
                    n144 = call "Elapsed Time"("Time Target (s)"=w385, "Reset"=w384, "Auto Reset"=FALSE) -> ("Time has Elapsed"=w382:bool)  [unwired: 9 in, 7 out]
                    n145 = And(x=w378, y=w363) -> (x .and. y?=w365:bool)
                    n146 = Select(t="Set rif vel" ("f"), s=w365, f=w379) -> (s? t:f=w377:string)
                    n147 = Select(t=w379, s=w364, f=w377) -> (s? t:f=w386:string)
                  }
                  frame "Set rif vel" {
                    # "set AO rif vel freno"
                    n148 = Subtract(x=w404, y=w405) -> (x-y=w403:dbl)
                    n149 = Greater?(x=w404, y=w405) -> (0:w413:bool)
                    n150 = Divide(x=w403, y=w402) -> (x/y=w401:dbl)
                    n151 = Multiply(x=w401, y=w397) -> (x*y=w400:dbl)
                    n152 = local read "RPM iniziali"() -> (w411:dbl)
                    n153 = Multiply(x=5.0, y=w397) -> (x*y=w398:dbl)
                    n154 = Absolute Value(x=w400) -> (abs(x)=w395:dbl)
                    n155 = In Range and Coerce(upper limit=w398, x=w395, lower limit=w397) -> (coerced(x)=w396:dbl)  [unwired: 1 out]
                    n156 = Multiply(x=w396, y=-1.0) -> (x*y=w406:dbl)
                    n157 = Select(t=w406, s=w413, f=w396) -> (s? t:f=w421:dbl)
                    n158 = Add(x=w421, y=w422) -> (x+y=w420:dbl)
                    n159 = Subtract(x=w411, y=w409) -> (x-y=w410:dbl)
                    n160 = Add(x=w409, y=w411) -> (x+y=w391:dbl)
                    n161 = In Range and Coerce(upper limit=4000.0, x=w391, lower limit=0.0) -> (coerced(x)=w388:dbl)  [unwired: 1 out]
                    n162 = In Range and Coerce(upper limit=w388, x=w420, lower limit=w410) -> (coerced(x)=w387:dbl)  [unwired: 1 out]
                    n163 = Divide(x=w387, y=w414) -> (x/y=w418:dbl)
                    n164 = Multiply(x=w418, y=100.0) -> (x*y=w416:dbl)
                    n165 = In Range and Coerce(upper limit=100.0, x=w416, lower limit=0.0) -> (coerced(x)=w407:dbl)  [unwired: 1 out]
                    n166 = Bundle By Name(cluster=T9 {"AO"=enum."*Rif vel inv freno", "Value"=0.0} ("Cluster SET AO"), "Value"=w407) -> (w393:T9)
                    n167 = Build Array(w393) -> (w392:T9[])
                    n168 = call "SET AO.vi"("Cluster SET AO"=w392) -> ()  [unwired: 10 in, 1 out]
                  }
                }
                n169 = property class="Clust (strict)"(reference=w336) -> (reference out=w334:refnum<vi>, "Value"=w335:cluster{"SET RPM":dbl, "SENSO ROT.":bool})  [unwired: 1 in, 1 out]
                n170 = Bundle By Name(cluster=w335, "SET RPM"=w332) -> (w333:cluster{"SET RPM":dbl, "SENSO ROT.":bool})
                n171 = property class="Clust (strict)"(reference=w334, "Value"=w333) -> ()  [unwired: 1 in, 2 out]
              }
              frame True {
                w461 = TRUE
                # "RAMPA PER EVITARE VARIAZIONI BRUSCHE"
                n172 = Not A Number/Path/Refnum?(number/path/refnum=w427) -> (NaN/Path/Refnum?=w428:bool)
                n173 = property class="Clust (strict)"(reference=w459) -> ("Value"=w460:cluster{"SET RPM":dbl, "SENSO ROT.":bool})  [unwired: 1 in, 2 out]
                n174 = local read "Ramp"() -> (w435:dbl[])
                n175 = Select(t=0.0, s=w428, f=w427) -> (s? t:f=w426:dbl)
                n176 = Equal?(x=FALSE, y=w455) -> (x = y?=w443:bool)
                n177 = Empty Array?(array=w435) -> (empty?=w434:bool)
                n178 = Delete From Array(array=w435, length=1, index=0) -> (deleted portion=w447:dbl[], array with subset deleted=w448:dbl[])
                n179 = feedback #3() -> (w458:dbl)  [unwired: 1 in]
                n180 = Not(x=w434) -> (.not. x?=w433:bool)
                n181 = Unbundle By Name(w460) -> ("SET RPM"=w445:dbl)
                n182 = Subtract(x=w445, y=w426) -> (x-y=w453:dbl)
                n183 = Absolute Value(x=w453) -> (abs(x)=w452:dbl)
                n184 = Quotient & Remainder(x=w452, y=100.0) -> (floor(x/y)=w432:dbl)  [unwired: 1 out]
                n185 = Index Array(array=w447) -> (element=w437:dbl)  [unwired: 1 in]
                n186 = feedback-in #3(w437) -> ()
                n187 = Not Equal?(x=w458, y=w437) -> (x != y?=w441:bool)
                n188 = In Range and Coerce(upper limit=50.0, x=w432, lower limit=2.0) -> (coerced(x)=w431:dbl)  [unwired: 1 out]
                n189 = local write "Ramp"(w448) -> ()
                n190 = Not A Number/Path/Refnum?(number/path/refnum=w437) -> (NaN/Path/Refnum?=w442:bool)
                n191 = Not(x=w442) -> (.not. x?=w440:bool)
                n192 = feedback #4() -> (w446:dbl)  [unwired: 1 in]
                n193 = feedback-in #4(w445) -> ()
                n194 = Compound Arithmetic op=AND(w441, w440, w433) -> (w439:bool)
                n195 = Not Equal?(x=w446, y=w445) -> (x != y?=w444:bool)
                n196 = case shown="True" w439 {
                  tunnel: w457 -> [_ w469]
                  tunnel: w437 -> [_ w468]
                  tunnel: [w467 w468] -> w436
                  tunnel: w426 -> [w467 _]
                  frame False {
                  }
                  frame True {
                    # "set AO rif vel freno"
                    n197 = Divide(x=w468, y=w469) -> (x/y=w477:dbl)
                    n198 = Multiply(x=w477, y=100.0) -> (x*y=w475:dbl)
                    n199 = In Range and Coerce(upper limit=100.0, x=w475, lower limit=-100.0) -> (coerced(x)=w470:dbl)  [unwired: 1 out]
                    n200 = Bundle By Name(cluster=T9 {"AO"=enum."*Rif vel inv freno", "Value"=0.0} ("Cluster SET AO"), "Value"=w470) -> (w472:T9)
                    n201 = Build Array(w472) -> (w471:T9[])
                    n202 = call "SET AO.vi"("Cluster SET AO"=w471) -> ()  [unwired: 10 in, 1 out]
                  }
                }
                n203 = Or(x=w443, y=w444) -> (x .or. y?=w438:bool)
                n204 = case shown="True" w438 {
                  tunnel: w426 -> [_ w463]
                  tunnel: w431 -> [_ w466]
                  tunnel: w445 -> [_ w464]
                  frame False {
                  }
                  frame True {
                    n205 = call-poly <vilib>:"Ramp Pattern.vi"("start"=w463, "end"=w464, "samples"=w466) -> ("Ramp Pattern"=→"Ramp":dbl[])  [unwired: 7 in, 1 out]
                  }
                }
                n206 = property class="DigNum (strict)"(reference=w424, "Value"=w423) -> ()  [unwired: 1 in, 2 out]
                n207 = local write "RPM iniziali"(w445) -> ()
              }
            }
          }
          frame True {
            w484 = 0.001 ("y")
            n208 = Unbundle By Name(w501) -> ("Vel max(RPM)"=w500:dbl)
            n209 = Unbundle By Name(w511) -> ()  [unwired: 1 out]
            n210 = global read "Servo avviamento.vi" "Cmecc con servo avviam"() -> (w485:bool)
            n211 = global read "Global_scelta_banco.vi" "banco 1?"() -> (w492:bool)
            n212 = Select(t="PID b1 gains ctrl velocità", s=w492, f="PID b2 gains ctrl velocità") -> (s? t:f=w490:T1)
            n213 = Divide(x=w514, y=u32 1000) -> (x/y=w512:dbl)
            n214 = call-poly <vilib>:"PID.vi"("reinitialize? (F)"="reinitialize? (F)", "output range"=cluster{"output high":dbl, "output low":dbl} {"output high"=2500.0, "output low"=-2500.0}, "dt (s)"=w512, "PID gains"=w490, "process variable"=w510, "setpoint"=w483) -> ("output"=w515:dbl)  [unwired: 4 in, 1 out]
            n215 = Multiply(x=w515, y=-1.0) -> (x*y=w494:dbl)
            n216 = Select(t=0.0, s="reinitialize? (F)", f=w494) -> (s? t:f=w486:dbl)
            n217 = Add(x=w507, y=w486) -> (x+y=w499:dbl)
            n218 = Divide(x=w499, y=w500) -> (x/y=w505:dbl)
            n219 = Add(x=w483, y=w484) -> (x+y=w509:dbl)
            n220 = Subtract(x=w483, y=w484) -> (x-y=w508:dbl)
            n221 = Multiply(x=w505, y=100.0) -> (x*y=w503:dbl)
            n222 = In Range and Coerce(upper limit=w509, x=w510, lower limit=w508) -> (In Range?=w488:bool)  [unwired: 1 out]
            n223 = Or(x=w488, y=w485) -> (x .or. y?=w487:bool)
            n224 = In Range and Coerce(upper limit=100.0, x=w503, lower limit=0.0) -> (coerced(x)=w498:dbl)  [unwired: 1 out]
            n225 = case shown="False" w487 {
              tunnel: w498 -> [w518 _]
              frame False {
                n226 = Bundle By Name(cluster=T9 {"AO"=enum."*Rif vel inv freno", "Value"=0.0} ("Cluster SET AO"), "Value"=w518) -> (w520:T9)
                n227 = Build Array(w520) -> (w521:T9[])
                n228 = call "SET AO.vi"("Cluster SET AO"=w521) -> ()  [unwired: 10 in, 1 out]
              }
              frame True {
              }
            }
          }
        }
        n229 = local write "reinitialize? (F)"(w278) -> ()
        n230 = global read "Global_scelta_banco.vi" "banco 1?"() -> (w276:bool)
        n231 = Or(x=w269, y=w291) -> (x .or. y?=w270:bool)
        n232 = Select(t=w277, s=w276, f=2.0) -> (s? t:f=w275:dbl)
        n233 = Select(t=w292, s=w270, f="Imposta controllo coppia" ("t")) -> (s? t:f=w293:string)
      }
      frame "Imposta controllo coppia" {
        w530 = 0.35  # isteresi min
        n234 = Unbundle By Name(w544) -> ("Cmax (nm)"=w543:dbl)
        n235 = Unbundle By Name(w534) -> ("statoAO_PLC.Rif vel freno"=w533:dbl, "statoAO_PLC.Rif coppia freno"=w532:dbl)
        n236 = Not A Number/Path/Refnum?(number/path/refnum=w524) -> (NaN/Path/Refnum?=w526:bool)
        n237 = Select(t=0.0, s=w526, f=w524) -> (s? t:f=w523:dbl)
        n238 = case shown="\"Fine imposta controllo coppia\"" w545 {
          selector: w545 -> [w551 w575 w586]
          tunnel: w543 -> [w562 _ _]
          tunnel: w523 -> [w561 w581 w584]
          tunnel: [w552 w573 w586] -> w542
          tunnel: [_ _ TRUE] -> w541
          tunnel: [w561 w581 w584] -> w537
          tunnel: w533 -> [_ w571 _]
          tunnel: w532 -> [w560 _ _]
          tunnel: w522 -> [w547 _ w582]
          frame "Set rif coppia", Default {
            # "set AO coppia"
            n239 = Multiply(x=w561, y=100.0) -> (x*y=w567:dbl)
            n240 = property class="DigNum (strict)"(reference=w547, "DisabledEnum"=T11."Disabled and Grayed Out" ("Disabled")) -> ()  [unwired: 1 in, 2 out]
            n241 = Divide(x=w567, y=w562) -> (x/y=w566:dbl)
            n242 = In Range and Coerce(upper limit=400.0, x=w566, lower limit=0.0) -> (coerced(x)=w556:dbl)  [unwired: 1 out]
            n243 = Multiply(x=0.99, y=w556) -> (x*y=w559:dbl)
            n244 = Multiply(x=1.01, y=w556) -> (x*y=w557:dbl)
            n245 = Bundle By Name(cluster=T9 {"AO"=enum."*Rif coppia inv freno", "Value"=0.0} ("Cluster SET AO"), "Value"=w556) -> (w550:T9)
            n246 = In Range and Coerce(upper limit=w557, x=w560, lower limit=w559) -> (In Range?=w554:bool)  [unwired: 1 out]
            n247 = Build Array(w550) -> (w548:T9[])
            n248 = call "SET AO.vi"("Cluster SET AO"=w548) -> ()  [unwired: 10 in, 1 out]
            n249 = Select(t="Set rif vel a 0", s=w554, f=w551) -> (s? t:f=w552:string)
          }
          frame "Set rif vel a 0" {
            w572 = 0.0 ("Value")
            # "set AO rif coppia a 0"
            n250 = Bundle By Name(cluster=T9 {"AO"=enum."*Rif vel inv freno", "Value"=0.0} ("Cluster SET AO"), "Value"=w572) -> (w570:T9)
            n251 = Multiply(x=0.99, y=w572) -> (x*y=w580:dbl)
            n252 = Multiply(x=1.01, y=w572) -> (x*y=w578:dbl)
            n253 = In Range and Coerce(upper limit=w578, x=w571, lower limit=w580) -> (In Range?=w576:bool)  [unwired: 1 out]
            n254 = Build Array(w570) -> (w568:T9[])
            n255 = call "SET AO.vi"("Cluster SET AO"=w568) -> ()  [unwired: 10 in, 1 out]
            n256 = Select(t="Fine imposta controllo coppia", s=w576, f=w575) -> (s? t:f=w573:string)
          }
          frame "Fine imposta controllo coppia" {
            n257 = property class="DigNum (strict)"(reference=w582, "DisabledEnum"=T11."Enabled" ("Disabled")) -> ()  [unwired: 1 in, 2 out]
          }
        }
        n258 = global read "Global_scelta_banco.vi" "banco 1?"() -> (w531:bool)
        n259 = global write "Global_Cmecc_RotBlocc.vi" "Cmecc/Rot blocc?"(FALSE ("Cmecc/Rot blocc?")) -> ()
        n260 = Select(t="Controllo coppia", s=w541, f=w540) -> (s? t:f=w539:string)
        n261 = Select(t=w530, s=w531, f=3.5) -> (s? t:f=w529:dbl)
      }
      frame "Verifica servo avviamento" {
        # "attendi che si stabilizzi\nla velocità di avvio impostata\nprima di passare\nin controllo di velocità"
        n262 = global read "Servo avviamento.vi" "Servo avviamento KO"() -> (w601:bool)
        n263 = global read "Servo avviamento.vi" "Servo avviamento ok"() -> (w598:bool)
        n264 = Not(x=w598) -> (.not. x?=w599:bool)
        n265 = Not(x=w601) -> (.not. x?=w600:bool)
        n266 = And(x=w600, y=w599) -> (x .and. y?=w591:bool)
        n267 = call "Elapsed Time6"("Time Target (s)"=3.0, "Reset"=w591, "Auto Reset"=FALSE) -> ("Time has Elapsed"=w590:bool)  [unwired: 9 in, 7 out]
        n268 = Select(t="Imposta controllo velocità", s=w598, f="Controllo coppia") -> (s? t:f=w588:string)
        n269 = Select(t=w588, s=w590, f=w589) -> (s? t:f=w595:string)
      }
    }
    n270 = Unbundle By Name(w79) -> ("Tempo rampa (s)"=w78:dbl)
    n271 = global write "Global stato ctrl coppia.vi" "controllo velocita?"(w76) -> ()
  }
  "Out C" <- w14
  "Tempo rampa (s)" <- w24
  "C stabile" <- w23
  "fine rampa C out" <- w22
  "Set C out" <- w3
